vi "elvisv1_2.vi"(0 "DeviceName":string, 1 "Amplitude":dbl, 2 "DC Offset":dbl, 3 "Frequency":dbl, 4 "Waveform Type":enum16{"Sine", "Triangular", "Square"}(ring), 5 "Sample Rate (Hz)":dbl=100000.0 caption="Sample rate (S/s)" min=0.0 step=1000000.0 format="%#_4p", 6 "Record Length":i32=2000 caption="Record length" min=5 max=75000000 step=1 format="%#.9p", 7 "Acquire":u16(ring)=10178 items=["N Samples"=10178, "Continuously"=10123], 8 "ChA_Source":T2 caption="Source" items=["BNC/Board CH A", "ACH0", "ACH1", "ACH2", "ACH5", "FGEN FUNC_OUT", "FGEN SYNC_OUT", "DMM Voltage"], 9 "ChB_Source":T1 caption="Source" items=["BNC/Board CH B", "ACH0", "ACH1", "ACH2", "ACH5", "FGEN FUNC_OUT", "FGEN SYNC_OUT", "DMM Voltage"], 10 "ChA Coupling":u16(ring) caption="Coupling" items=["DC", "AC"], 11 "ChB_ Coupling":u16(ring) caption="Coupling" items=["DC", "AC"], 12 "ChA Range":dbl caption="Range", 13 "ChB Range":dbl caption="Range", 14 "ChA Offset":dbl caption="Offset", 15 "ChB Offset":dbl caption="Offset", 16 "Trigger Source":u16(ring) caption="Source" items=["Immediate", "TRIGGER", "SYNC_OUT", "CH A", "CH B"], 17 "Trigger Type":u16(ring) caption="Type" items=["Digital", "Analog"], 18 "Slope":i32(ring) items=["Positive", "Negative"]) -> (22 "interleaved array":dbl[](array[numeric]))   [LabVIEW 2010]
uses:
  <instrlib>/NI ELVIS Traditional/NI ELVIS - Scope.llb/ELVIS SCOPE - Channel A Source.ctl
  <instrlib>/NI ELVIS Traditional/NI ELVIS - Scope.llb/ELVIS SCOPE - Channel B Source.ctl
panel:
  out "Device Name Indicator":tag="Dev1"
  in  "Device Name":tag="Dev1"
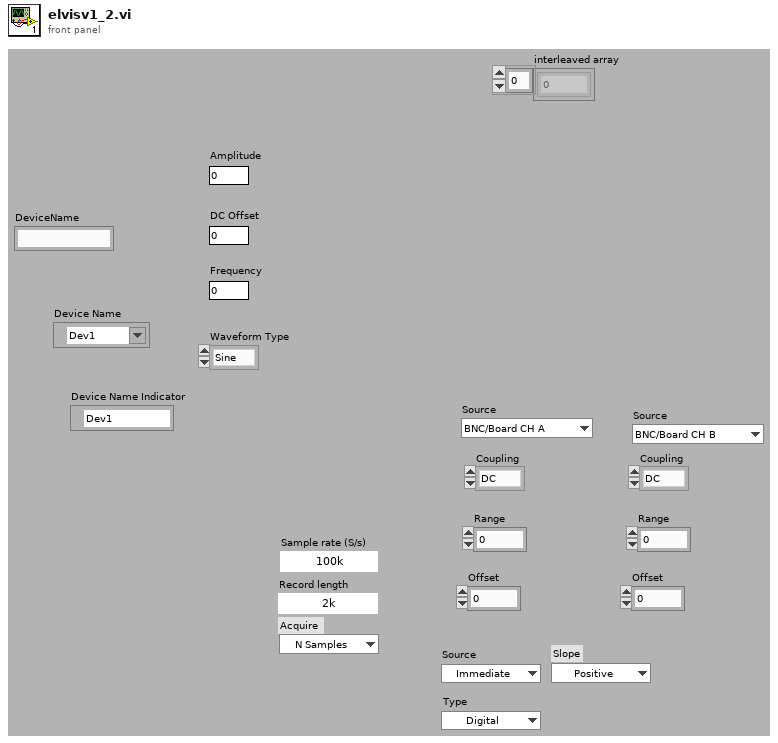
[diagram p1: front panel]
types:
  T1 = typedef "ELVIS SCOPE - Channel B Source.ctl" = u16
  T2 = typedef "ELVIS SCOPE - Channel A Source.ctl" = u16
  T3 = typedef "ELVIS RSCMAN - NI ELVIS Refnum.ctl" = refnum<k1>
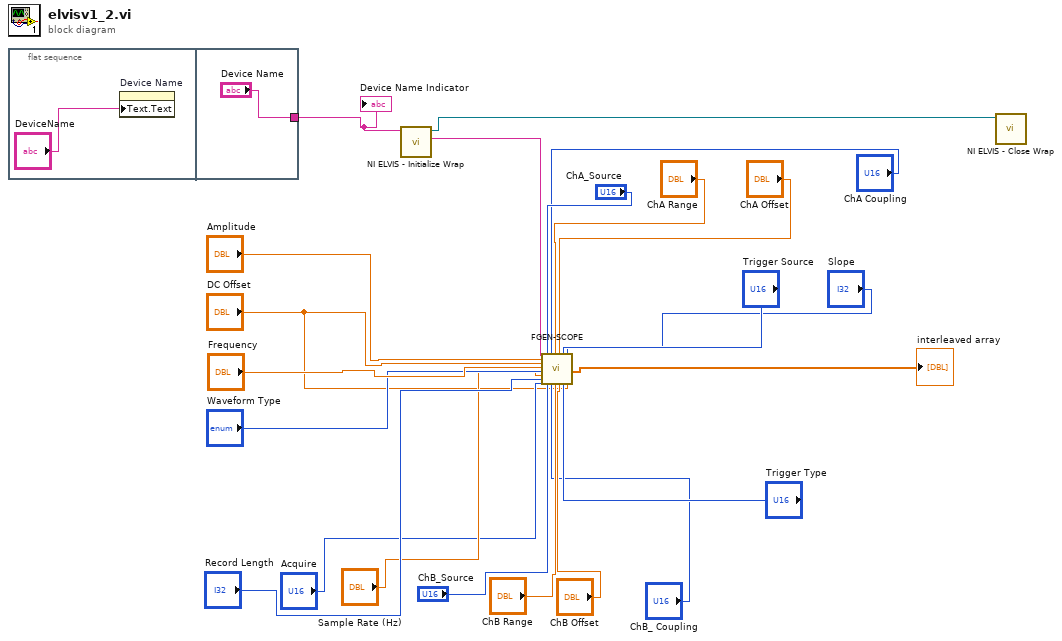
[diagram p0: block diagram]
diagram:
  n1 = flat-sequence {
    tunnel: ["Device Name"] -> w1
    frame #0 {
      n2 = property on="Device Name" class="DAQmxName"("Text.Text"="DeviceName") -> ()  [unwired: 2 in, 2 out]
    }
    frame #1 {
    }
  }
  n3 = call "NI ELVIS - Initialize Wrap.vi"("Device Name"=w1) -> ("Device Name (out)"=w4:tag, "NI ELVIS Refnum"=w3:T3)  [unwired: 8 in, 1 out]
  n4 = call "FGEN-SCOPE.vi"("Device Name"=w4, "Amplitude"="Amplitude", "DC Offset"="DC Offset", "Frequency"="Frequency", "Waveform Type"="Waveform Type", "Sample Rate (Hz)"="Sample Rate (Hz)", "Record Length"="Record Length", "Acquire"="Acquire", "ChA_Source"="ChA_Source", "ChB_Source"="ChB_Source", "ChA Coupling"="ChA Coupling", "ChB_ Coupling"="ChB_ Coupling", "ChA Range"="ChA Range", "ChB Range"="ChB Range", "ChA Offset"="ChA Offset", "ChB Offset"="ChB Offset", "Trigger Source"="Trigger Source", "Trigger Type"="Trigger Type", "Slope"="Slope", "Level"="DC Offset") -> ("interleaved array"=→"interleaved array":dbl[])  [unwired: 6 in, 1 out]
  n5 = call "NI ELVIS - Close Wrap.vi"("NI ELVIS Refnum In"=w3) -> ()  [unwired: 10 in, 1 out]
  "Device Name Indicator" <- w1
